vi "Position Window.vi"(8 "error in (no error)":errorcluster, 10 "Force Reposition?":bool, 11 "Window in":refnum<class "Window.lvclass">) -> (0 "error out":errorcluster)   [LabVIEW 2017, in "MGI-Panel Manager.lvlib" / "Window.lvclass"]
doc: "Repositions the window according the the configured window positions.\n\nIf <b>Force Reposition?</b> is false, then the window will only be repositioned if the front panel was previously not shown.\nIf <b>Force Reposition?</b> is true, then the window will be repositioned regardless of the front panel's state.\n\n----\nPlease see the following web address for additional documentation and tutorial information:\nhttp://www.mooregoodideas.com/mgi-panel-manager/\n\nAuthor: Derek Trepanier\n\nCopyright (c) 2018, Moore Good Ideas, Inc.\n\nAll rights reserved.\n\nRedistribution and use in source and binary forms, with or without modification, are permitted provided that the following conditions are met:\n\n * Redistributions of source code must retain the above copyright notice, this list of conditions and the following disclaimer.\n * Redistributions in binary form must reproduce the above copyright notice, this list of conditions and the following disclaimer in the documentation and/or other materials provided with the distribution.\n * Neither the name of Moore Good Ideas, Inc. nor the names of its contributors may be used to endorse or promote products derived from this software without specific prior written permission.\n\nTHIS SOFTWARE IS PROVIDED BY THE COPYRIGHT HOLDERS AND CONTRIBUTORS \"AS IS\" AND ANY EXPRESS OR IMPLIED WARRANTIES, INCLUDING, BUT NOT LIMITED TO, THE IMPLIED WARRANTIES OF MERCHANTABILITY AND FITNESS FOR A PARTICULAR PURPOSE ARE DISCLAIMED. IN NO EVENT SHALL THE COPYRIGHT OWNER OR CONTRIBUTORS BE LIABLE FOR ANY DIRECT, INDIRECT, INCIDENTAL, SPECIAL, EXEMPLARY, OR CONSEQUENTIAL DAMAGES (INCLUDING, BUT NOT LIMITED TO, PROCUREMENT OF SUBSTITUTE GOODS OR SERVICES; LOSS OF USE, DATA, OR PROFITS; OR BUSINESS INTERRUPTION) HOWEVER CAUSED AND ON ANY THEORY OF LIABILITY, WHETHER IN CONTRACT, STRICT LIABILITY, OR TORT (INCLUDING NEGLIGENCE OR OTHERWISE) ARISING IN ANY WAY OUT OF THE USE OF THIS SOFTWARE, EVEN IF ADVISED OF THE POSSIBILITY OF SUCH DAMAGE."
uses:
  Window.lvclass
  D:/software/LabView_PanelManager/panel-manager/Source/Panel/Panel.lvclass
  Panel.lvclass/Panel.ctl
  Window.lvclass/Window.ctl
  Window Position/Window Position.lvclass
  Panel.lvclass
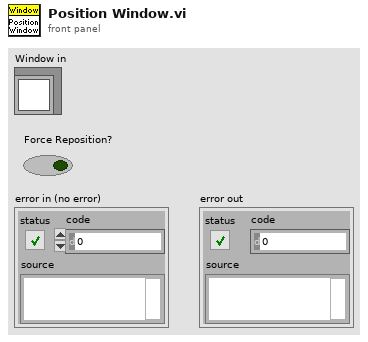
[diagram p1: front panel]
types:
  T1 = enum32{"Invalid", "Standard", "Closed", "Hidden", "Minimized", "Maximized"}[]
  T2 = enum32{"Invalid", "Standard", "Closed", "Hidden", "Minimized", "Maximized"}
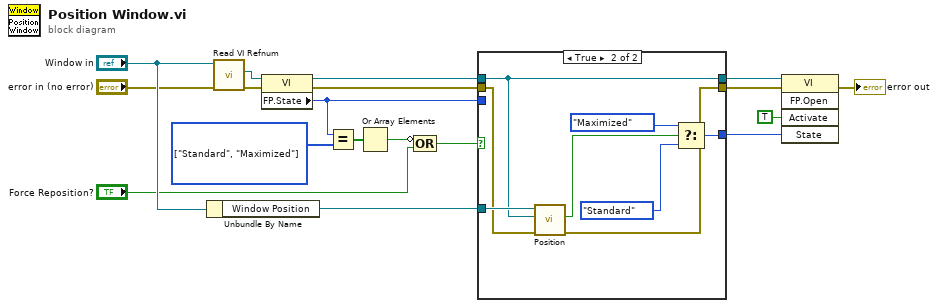
[diagram p0: block diagram]
diagram:
  w6 = T1 [enum."Standard", enum."Maximized"] items=["Invalid", "Standard", "Closed", "Hidden", "Minimized", "Maximized"]
  n1 = Unbundle By Name("Window in") -> ("Window Position"=w8:refnum<class "Window Position.lvclass">)
  n2 = call "Read VI Refnum.vi"("error in (no error)"="error in (no error)", "Panel in"="Window in") -> ("error out"=w7:errorcluster, "VI Refnum"=w12:refnum<vi>)  [unwired: 8 in]
  n3 = property class="VI"(reference=w12, error in=w7) -> (reference out=w13:refnum<vi>, error out=w11:errorcluster, "FP.State"=w5:T2)
  n4 = Equal?(x=w5, y=w6) -> (x = y?=w4:bool[])
  n5 = Or Array Elements(Boolean array=w4) -> (logical OR=w3:bool)
  n6 = Compound Arithmetic op=OR(invert w3, "Force Reposition?") -> (w1:bool)
  n7 = case shown="True" w1 {
    tunnel: w11 -> [w21 w28]
    tunnel: w13 -> [w20 w26]
    tunnel: [w21 w27] -> w16
    tunnel: w8 -> [_ w29]
    tunnel: [w20 w26] -> w15
    tunnel: [w19 w22] -> w18
    tunnel: w5 -> [w19 _]
    frame False {
    }
    frame True {
      n8 = call-dynamic "Position.vi"("error in (no error)"=w28, "Panel VI"=w26, "Window Position in"=w29) -> ("error out"=w27:errorcluster, "Open Maximized?"=w25:bool)  [unwired: 7 in]
      n9 = Select(t=T2."Maximized" ("FP.State"), s=w25, f=T2."Standard" ("FP.State")) -> (s? t:f=w22:T2)
    }
  }
  n10 = invoke class="VI" method="FP.Open"(reference=w15, error in=w16, "Activate"=TRUE ("Activate?"), "State"=w18) -> (error out=→"error out":errorcluster)  [unwired: 1 in, 4 out]
